vi "WriteDLP2Config.vi"(8 "error in (no error)":errorcluster, 10 "MasterConfigurationDLPC2":T1={"Paths"={"DigiBit WG Design Folder"=path "C:/projects/Digilens_IPLC", "Compensated GS Image Folder"=path "C:/projects/Digilens_IPLC", "Nozzle GS Files Head 1"=path "C:/projects/Digilens_IPLC/DLPC2Config.xml", "Nozzle GS Files Head 2"=path "C:/projects/Digilens_IPLC/DLPC2Config.xml", "Nozzle GS Files Head 3"=path "C:/projects/Digilens_IPLC/DLPC2Config.xml", "Nozzle GS Files Head 4"=path "C:/projects/Digilens_IPLC/DLPC2Config.xml", "Nozzle GS Files Head 5"=path "C:/projects/Digilens_IPLC/DLPC2Config.xml", "Nozzle GS Files Head 6"=path "C:/projects/Digilens_IPLC/DLPC2Config.xml"}, "ColorPaneMapping"={"Head 1"={"Material"="109G", "ColorPane"="0-C"}, "Head 2"={"Material"="311A", "ColorPane"="1-M"}, "Head 3"={"Material"="FD/OP-3", "ColorPane"="2-Y"}, "Head 4"={"Material"="311A", "ColorPane"="3-K"}, "Head 5"={"Material"="507 - 100%", "ColorPane"="4-Blue-Spot"}, "Head 6"={"Material"="507 - 50%", "ColorPane"="5-Orange-Spot"}}, "Materials"=["109G", "311A", "FD/OP-3", "507 - 100%", "507 - 50%"], "ColorPlanes"=["0-C", "1-M", "2-Y", "3-K", "4-Blue-Spot", "5-Orange-Spot"], "SpitVoltages_Half"={"1"=0.0, "2"=0.0, "3"=0.0, "4"=0.0, "5"=0.0, "6"=0.0}, "SpitVoltages_Full"={"1"=0.0, "2"=0.0, "3"=0.0, "4"=0.0, "5"=0.0, "6"=0.0}, "SystemMode"=[], "PrimeModeConfig"=[]}, 11 "XML File Path":path) -> (0 "error out":errorcluster, 3 "XML File Path (duplicate)":path)   [LabVIEW 2022 SP3]
uses:
  Controls/TD MasterConfiguration DLPC2--cluster.ctl
  Controls/DLPC2_Path--Cluster.ctl
  Controls/TD HeadColorPaneMappingAll--cluster.ctl
  Controls/TD HeadColorPaneMapping--cluster.ctl
  Classes/TopLevel/Typedefs/SpitVoltages--Cluster.ctl
  Classes/TopLevel/Typedefs/PrimingMode APIData.ctl
  Classes/TopLevel/Typedefs/PurgeMode--Enum.ctl
  Classes/TopLevel/Typedefs/PrinterHeads--Enum.ctl
  Classes/TopLevel/TopLevel.lvclass
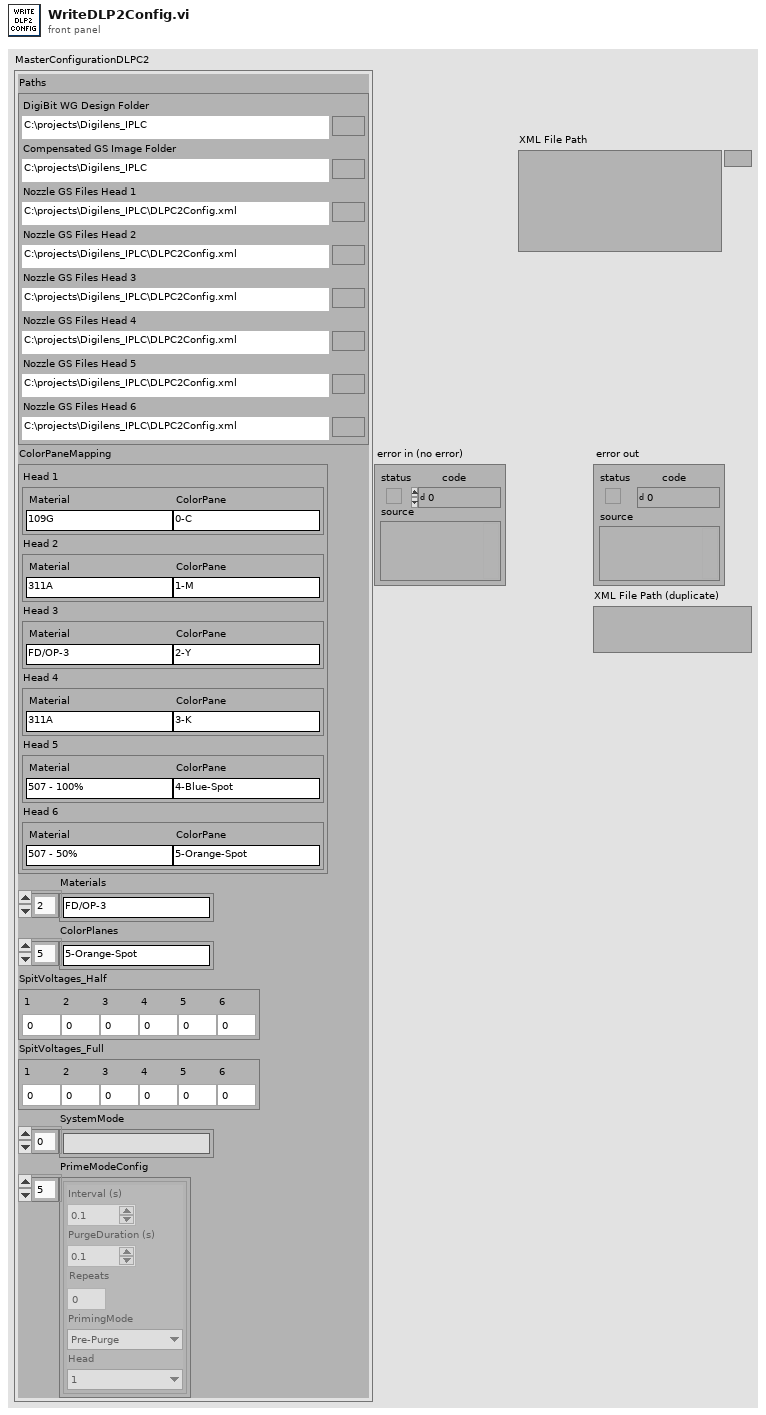
[diagram p1: front panel]
types:
  T1 = typedef "TD MasterConfiguration DLPC2--cluster.ctl" = cluster{"Paths":T2, "ColorPaneMapping":T3, "Materials":string[], "ColorPlanes":string[], "SpitVoltages_Half":T5, "SpitVoltages_Full":T5, "SystemMode":string[], "PrimeModeConfig":T6[]}
  T2 = typedef "DLPC2_Path--Cluster.ctl" = cluster{"DigiBit WG Design Folder":path, "Compensated GS Image Folder":path, "Nozzle GS Files Head 1":path, "Nozzle GS Files Head 2":path, "Nozzle GS Files Head 3":path, "Nozzle GS Files Head 4":path, "Nozzle GS Files Head 5":path, "Nozzle GS Files Head 6":path}
  T3 = typedef "TD HeadColorPaneMappingAll--cluster.ctl" = cluster{"Head 1":T4, "Head 2":T4, "Head 3":T4, "Head 4":T4, "Head 5":T4, "Head 6":T4}
  T4 = typedef "TD HeadColorPaneMapping--cluster.ctl" = cluster{"Material":string, "ColorPane":string}
  T5 = typedef "SpitVoltages--Cluster.ctl" = cluster{"1":dbl, "2":dbl, "3":dbl, "4":dbl, "5":dbl, "6":dbl}
  T6 = typedef "TopLevel.lvclass/PrimingMode APIData.ctl" = cluster{"Interval (s)":dbl, "PurgeDuration (s)":dbl, "Repeats":u8, "PrimingMode":T7, "Head":T8}
  T7 = typedef "PurgeMode--Enum.ctl" = enum16{"Pre-Purge", "Purge", "Spit", "Prime"}
  T8 = typedef "PrinterHeads--Enum.ctl" = enum16{"1", "2", "3", "4", "5", "6", "-1"}
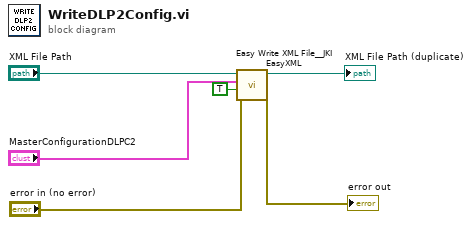
[diagram p0: block diagram]
diagram:
  n1 = call <vilib>:"Easy Write XML File__JKI EasyXML.vi"("error in (no error)"="error in (no error)", "Overwrite File? (false)"=TRUE, "LabVIEW Data"="MasterConfigurationDLPC2", "XML File Path"="XML File Path") -> ("error out"=→"error out":errorcluster, "XML File Path (duplicate)"=→"XML File Path (duplicate)":path)  [unwired: 6 in]
